vi "TC-01-(Acquire)CreateSavingCommand.vi"(8 "error in (no error)":errorcluster, 11 "NI-TC-01 in":refnum<class "NI-TC-01.lvclass">) -> (0 "error out":errorcluster, 2 "SavingCommand":string, 3 "NI-TC-01 out":refnum<class "NI-TC-01.lvclass">)   [LabVIEW 2020, in "NI-TC-01.lvclass"]
uses:
  NI-TC-01.lvclass
  NI-TC-01.lvclass/NI-TC-01.ctl
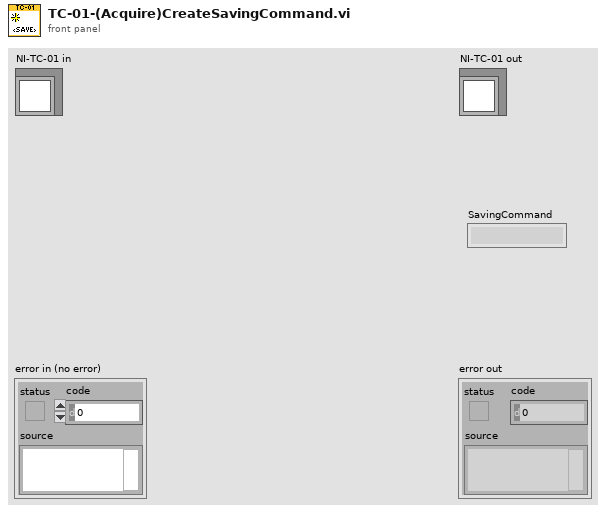
[diagram p1: front panel]
types:
  T1 = typedef "OnOffTypeDef.ctl" = enum16{"off", "on"}
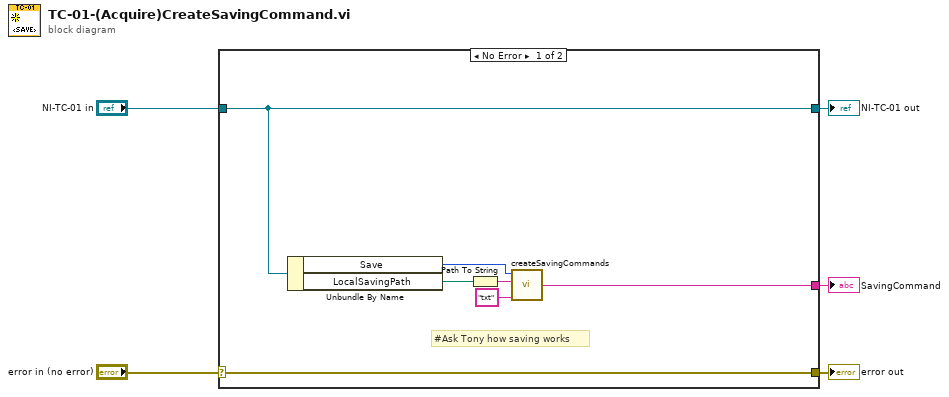
[diagram p0: block diagram]
diagram:
  n1 = case shown="No Error" "error in (no error)" {
    selector: "error in (no error)" -> [w12 w14]
    tunnel: [w12 w14] -> w4
    tunnel: [w9 w13] -> w2
    tunnel: "NI-TC-01 in" -> [w9 w13]
    tunnel: [w7 _] -> w1
    frame No Error {
      # "#Ask Tony how saving works"
      n2 = Unbundle By Name(w9) -> ("Save"=w6:T1, "LocalSavingPath"=w8:path)
      n3 = Path To String(path=w8) -> (string=w10:string)
      n4 = call "createSavingCommands.vi"("extension"="txt" ("Fileextension"), "Saving Path (local)"=w10, "Save"=w6) -> ("String"=w7:string)  [unwired: 1 in]
    }
    frame Error {
    }
  }
  "error out" <- w4
  "NI-TC-01 out" <- w2
  "SavingCommand" <- w1
